vi "I2C Close.vi"(7 "I2C Channel (0)":u8, 8 "Error In":errorcluster, 11 "LINX Resource":T1) -> (0 "Error Out":errorcluster, 3 "LINX Resource":T1)   [LabVIEW 2013, in "LVH-LINX.lvlib"]
doc: "Close the specified I2C channel."
uses:
  <vilib>/LabVIEW Hacker/LINX/LVH-LINX.lvlib
  <vilib>/LabVIEW Hacker/LINX/Private/Type Defs/LINX Ref.ctl
  <vilib>/LabVIEW Hacker/LINX/Private/Type Defs/Platform.ctl
  <vilib>/LabVIEW Hacker/LINX/Private/Type Defs/Interface.ctl
  <vilib>/LabVIEW Hacker/LINX/Private/Device/Type Defs/LINX Device Config.ctl
  <vilib>/LabVIEW Hacker/LINX/Private/Device/Type Defs/TCP Config.ctl
  <vilib>/LabVIEW Hacker/LINX/Private/Type Defs/Device Family.ctl
  <vilib>/LabVIEW Hacker/LINX/Private/Type Defs/Peripheral.ctl
  <vilib>/LabVIEW Hacker/LINX/Private/Type Defs/Channel FGV States.ctl
  <vilib>/myRIO/Instrument Drivers/Onboard IO/I2C/typedefs/I2C Transfer Rate.ctl
  <vilib>/myRIO/Instrument Drivers/Onboard IO/I2C/typedefs/I2C Configuration.ctl
  <vilib>/myRIO/Common/Instrument Driver Framework/myRIO v1.0/I2C/typedefs/I2C Channels Enum.ctl
  <vilib>/myRIO/Common/Instrument Driver Framework/Utilities/typedefs/Generic FPGA Reference.ctl
  <vilib>/myRIO/Common/Instrument Driver Framework/Utilities/typedefs/myRIO v1.0 Reference.ctl
  <vilib>/myRIO/Common/Instrument Driver Framework/Utilities/typedefs/Hardware Version Enum.ctl
  <vilib>/myRIO/Common/Instrument Driver Framework/Utilities/typedefs/myRIO Generic Hardware Reference.ctl
  <vilib>/myRIO/Instrument Drivers/Onboard IO/I2C/typedefs/I2C Reference.ctl
  <vilib>/LabVIEW Hacker/LINX/Private/Device/Device.lvlib
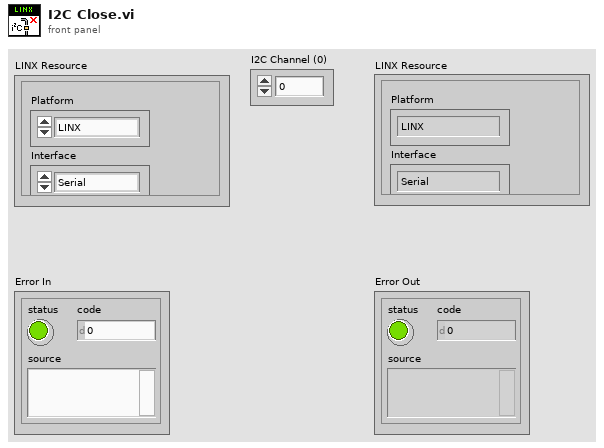
[diagram p1: front panel]
types:
  T1 = typedef "LVH-LINX.lvlib/LINX Ref.ctl" = cluster{"Platform":T2, "Interface":T3, "LINX Device Config":T4}
  T2 = typedef "LVH-LINX.lvlib/Platform.ctl" = enum16{"LINX", "myRIO"}
  T3 = typedef "LVH-LINX.lvlib/Interface.ctl" = enum16{"Serial", "TCP"}
  T4 = typedef "LVH-LINX.lvlib/Device.lvlib/LINX Device Config.ctl" = cluster{"Interface":T3, "COM Port":refnum<visa-resource-name>, "TCP Configuration":T5, "Device Family":T6, "Device ID":u8, "Device Name":string, "TCP Ref":refnum<k5>}
  T5 = typedef "LVH-LINX.lvlib/Device.lvlib/TCP Config.ctl" = cluster{"IP Address":string, "Port":u16}
  T6 = typedef "LVH-LINX.lvlib/Device Family.ctl" = enum8{"National Instruments", "Digilent", "Arduino"}
  T7 = typedef "LVH-LINX.lvlib/Peripheral.ctl" = enum8{"DI", "DO", "AI", "AO", "PWM", "QE", "UART", "I2C", "SPI", "CAN"}
  T8 = typedef "LVH-LINX.lvlib/Channel FGV States.ctl" = enum16{"Initialize", "Get", "Set"}
  T9 = typedef "I2C.lvlib/I2C Reference.ctl" = cluster{"myRIO Reference":T10, "I2C Channels Enum":T14, "I2C Configuration":T15}
  T10 = typedef "myRIO Generic Hardware Reference.ctl" = cluster{"myRIO Model":T11, "myRIO Hardware Reference":T12}
  T11 = typedef "Hardware Version Enum.ctl" = enum16{"Unknown", "myRIO-1900", "myRIO-1950"}
  T12 = typedef "myRIO v1.0 Reference.ctl" = cluster{"Generic FPGA Reference":T13, "Allow multiple opens":bool}
  T13 = typedef "Generic FPGA Reference.ctl" = refnum<k20>
  T14 = typedef "I2C Channels Enum.ctl" = enum16{"Not Connected", "A/I2C", "B/I2C"}
  T15 = typedef "I2C.lvlib/I2C Configuration.ctl" = cluster{"I2C Transfer Rate":T16}
  T16 = typedef "I2C.lvlib/I2C Transfer Rate.ctl" = enum16{"Standard Mode (100 kbps)", "Fast Mode (400 kbps)"}
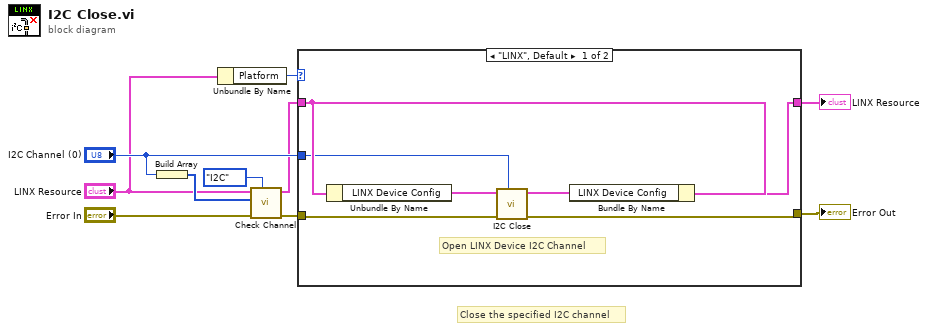
[diagram p0: block diagram]
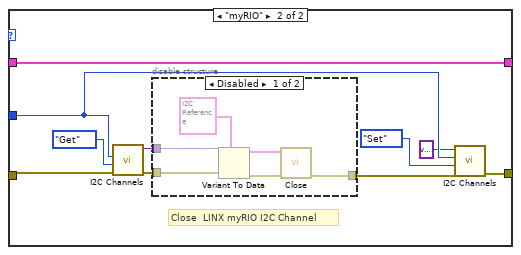
[diagram p2: hidden frame]
diagram:
  # "Close the specified I2C channel"
  n1 = Build Array("I2C Channel (0)") -> (w7:u8[])
  n2 = Unbundle By Name("LINX Resource") -> ("Platform"=w10:T2)
  n3 = call <vilib>:"Check Channel.vi"("Peripheral"=Peripheral."I2C", "Error In"="Error In", "Channels"=w7, "LINX Resource"="LINX Resource") -> ("Error Out"=w4:errorcluster, "LINX Resource"=w1:T1)  [unwired: 5 in, 1 out]
  n4 = case shown="\"LINX\", Default" w10 {
    tunnel: w4 -> [w12 w23]
    tunnel: w1 -> [w17 w27]
    tunnel: [w11 w26] -> w9
    tunnel: [w16 w27] -> w8
    tunnel: "I2C Channel (0)" -> [w13 w22]
    frame "LINX", Default {
      # "Open LINX Device I2C Channel"
      n5 = Unbundle By Name(w17) -> ("LINX Device Config"=w15:T4)
      n6 = call <vilib>:"I2C Close.vi"("I2C Channel"=w13, "Error In"=w12, "LINX Device Config"=w15) -> ("Error Out"=w11:errorcluster, "LINX Device Config"=w14:T4)  [unwired: 7 in]
      n7 = Bundle By Name(cluster=w17, "LINX Device Config"=w14) -> (w16:T1)
    }
    frame "myRIO" {
      # "Close  LINX myRIO I2C Channel"
      n8 = call <vilib>:"I2C Channels.vi"("Error In"=w23, "Channel State"=Channel_FGV_States."Get", "Channel Number"=w22) -> ("Error Out"=w20:errorcluster, "I2C Channel"=w21:variant)  [unwired: 7 in]
      n9 = disable-structure shown="Disabled" {
        disable-tunnel: w21 -> [w30 _]
        disable-tunnel: w20 -> [w29 _]
        disable-tunnel: [w28 _] -> w19
        frame Disabled {
          n10 = Variant To Data(error in=w29, type=T9 {"myRIO Reference"={"myRIO Model"=enum."Unknown", "myRIO Hardware Reference"={"Generic FPGA Reference"=refnum, "Allow multiple opens"=FALSE}}, "I2C Channels Enum"=enum."Not Connected", "I2C Configuration"={"I2C Transfer Rate"=enum."Standard Mode (100 kbps)"}}, Variant=w30) -> (data=w32:T9, error out=w31:errorcluster)
          n11 = call <vilib>:"Close.vi"("error in (no error)"=w31, "I2C Ref In"=w32) -> ("error out"=w28:errorcluster)  [unwired: 9 in]
        }
        frame Enabled {
        }
      }
      n12 = call <vilib>:"I2C Channels.vi"("Error In"=w19, "Channel State"=Channel_FGV_States."Set", "Channel Number"=w22, "I2C Channel"=variant) -> ("Error Out"=w26:errorcluster)  [unwired: 6 in, 1 out]
    }
  }
  "Error Out" <- w9
  "LINX Resource" <- w8
